vi "Read Identity.vi"() -> ()   [LabVIEW 2020, in "CTI-Visa-Scratchpad.lvlib"]
uses:
  CTI-Visa-Scratchpad.lvlib
  CTI-Visa/CTI-Visa.lvlib
  CTI-Visa/Identity.ctl
panel:
  out "Identity":T1
  out "error out":errorcluster
  in  "Port":refnum<visa-resource-name>="COM3"
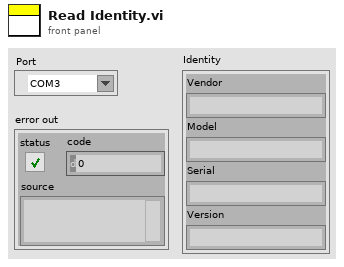
[diagram p1: front panel]
types:
  T1 = typedef "CTI-Visa.lvlib/Identity.ctl" = cluster{"Vendor":string, "Model":string, "Serial":string, "Version":string}
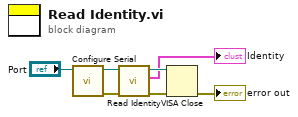
[diagram p0: block diagram]
diagram:
  n1 = call "Configure Serial.vi"("VISA resource name in"="Port") -> ("error out"=w5:errorcluster, "VISA resource name"=w6:refnum<visa-resource-name>)  [unwired: 9 in]
  n2 = call "Read Identity.vi"("error in (no error)"=w5, "VISA resource name in"=w6) -> ("error out"=w4:errorcluster, "Identity"=→"Identity":T1, "VISA resource name"=w2:refnum<visa-resource-name>)  [unwired: 7 in]
  n3 = VISA Close(VISA resource name=w2, error in (no error)=w4) -> (error out=→"error out":errorcluster)
